vi "Read Alarm Info.vi"(8 "error in (no error)":errorcluster, 10 "Node (3)":u8=3 caption="Node" min=3 max=128 step=1, 11 "VISA resource name":refnum<visa-resource-name>) -> (0 "error out":errorcluster, 2 "Alarm Message":string, 3 "VISA resource name out":refnum<visa-resource-name>)   [LabVIEW 2023, in "Bronkhorst FLOW-BUS.lvlib"]
doc: "Reads the value of alarm info that contains 8 bits with status information about some (alarm) events in the instrument. The 8 bit status is checked (as a hexadeciamal string) and the corresponding error is outputted."
uses:
  Bronkhorst FLOW-BUS.lvlib
  Private/FLOW-BUS RW.ctl
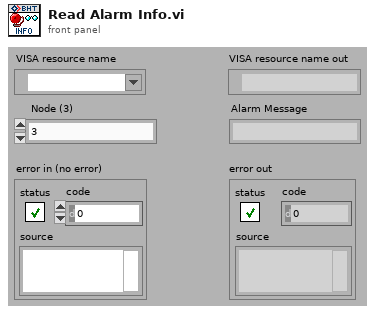
[diagram p1: front panel]
types:
  T1 = typedef "Bronkhorst FLOW-BUS.lvlib/FLOW-BUS RW.ctl" = cluster{"Node Address (3)":u8, "Communication Command":enum16{"Status message", "Send parameter with destination address and 00 response", "Send parameter with destination address", "Request parameter"}, "Process (0)":u16, "Parameter (0)":u16, "Data Type (0: Character)":enum16{"Character", "Integer", "Float or Long", "String"}, "Data for Char, Int, or Long (0)":u32, "Data for Float (0)":sgl, "Data for String":string, "Length of Requested String (0)":u8}
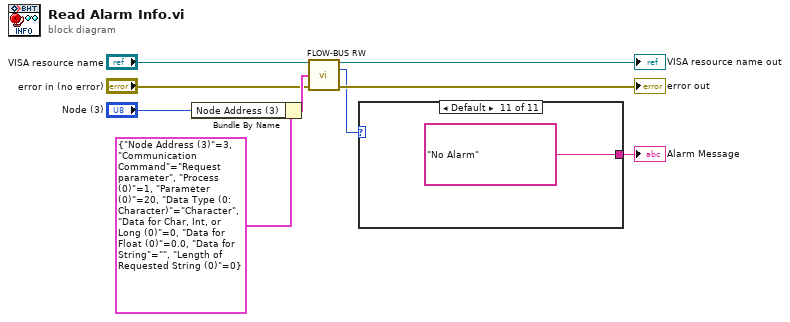
[diagram p0: block diagram]
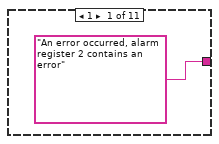
[diagram p2: hidden frame]
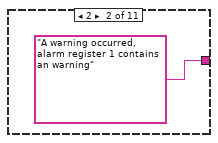
[diagram p3: hidden frame]
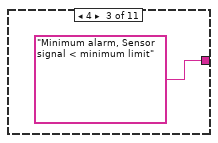
[diagram p4: hidden frame]
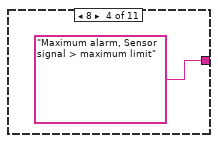
[diagram p5: hidden frame]
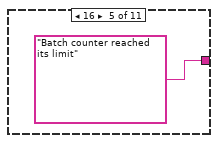
[diagram p6: hidden frame]
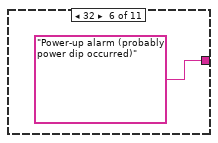
[diagram p7: hidden frame]
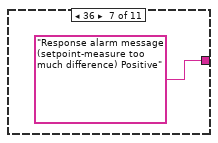
[diagram p8: hidden frame]
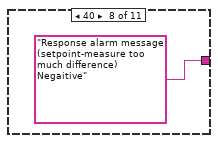
[diagram p9: hidden frame]
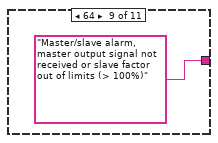
[diagram p10: hidden frame]
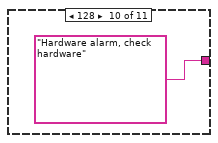
[diagram p11: hidden frame]
diagram:
  n1 = Bundle By Name(cluster=T1 {"Node Address (3)"=3, "Communication Command"=enum."Request parameter", "Process (0)"=1, "Parameter (0)"=20, "Data Type (0: Character)"=enum."Character", "Data for Char, Int, or Long (0)"=0, "Data for Float (0)"=0.0, "Data for String"="", "Length of Requested String (0)"=0} ("FLOW-BUS Command Settings"), "Node Address (3)"="Node (3)") -> (w8:T1)
  n2 = call "FLOW-BUS RW.vi"("VISA resource name"="VISA resource name", "FLOW-BUS Command Settings"=w8, "error in (no error)"="error in (no error)") -> ("VISA resource name out"=→"VISA resource name out":refnum<visa-resource-name>, "Requested Char, Int or Long"=w2:u32, "error out"=→"error out":errorcluster)  [unwired: 8 in, 2 out]
  n3 = case shown="Default" w2 {
    tunnel: ["An error occurred, alarm register 2 contains an error" ("write buffer (\"\")") "A warning occurred, alarm register 1 contains an warning" ("write buffer (\"\")") "Minimum alarm, Sensor signal < minimum limit" ("write buffer (\"\")") "Maximum alarm, Sensor signal > maximum limit" ("write buffer (\"\")") "Batch counter reached its limit" ("write buffer (\"\")") "Power-up alarm (probably power dip occurred)" ("write buffer (\"\")") "Response alarm message (setpoint-measure too much difference) Positive" ("write buffer (\"\")") "Response alarm message (setpoint-measure too much difference) Negaitive" ("write buffer (\"\")") "Master/slave alarm, master output signal not received or slave factor out of limits (> 100%)" ("write buffer (\"\")") "Hardware alarm, check hardware" ("write buffer (\"\")") "No Alarm" ("write buffer (\"\")")] -> w9
    frame 1 {
    }
    frame 2 {
    }
    frame 4 {
    }
    frame 8 {
    }
    frame 16 {
    }
    frame 32 {
    }
    frame 36 {
    }
    frame 40 {
    }
    frame 64 {
    }
    frame 128 {
    }
    frame Default {
    }
  }
  "Alarm Message" <- w9
